vi "test-new-clock-3.vi"() -> ()   [LabVIEW 2019]
uses:
  <vilib>/Rock Robotics/WPI/ThirdParty/JAS_Junk/TrajLib/Trajectory_Library.lvlib
  <vilib>/Utility/RT CPU Load.ctl
panel:
  out "Overflow count":i32
  out "Loop5":i32
  out "Err Sum6":i32
  out "Clock6":dbl
  out "Err Sum5":i32
  out "Clock5":dbl
  out "RoboRIO CPU loads":T1[](array[typedef]) {"ISR (%)" format="%#.2f"; "Idle (%)" format="%#.2f"; "Background (%)" format="%#.2f"; "Normal (%)" format="%#.2f"; "Above Normal (%)" format="%#.2f"; "High (%)" format="%#.2g"; "Timed Structures (%)" format="%#.2g"; "Time Critical (%)" format="%#.2g"; "Total (%)" format="%#.2g"}
  out "Diff":dbl
  out "Err Sum4":i32
  out "Clock4":dbl
  out "Err Sum3":i32
  out "Clock3":dbl
  out "Err Sum2":i32
  out "Clock2":dbl
  out "Clock1":dbl
  out "Err Sum1":i32
  out "OS Clock":dbl format="%35.6f"
  out "Error Count":i32
  out "Loop Count":i32
  out "FPGA Clock":dbl format="%35.6f"
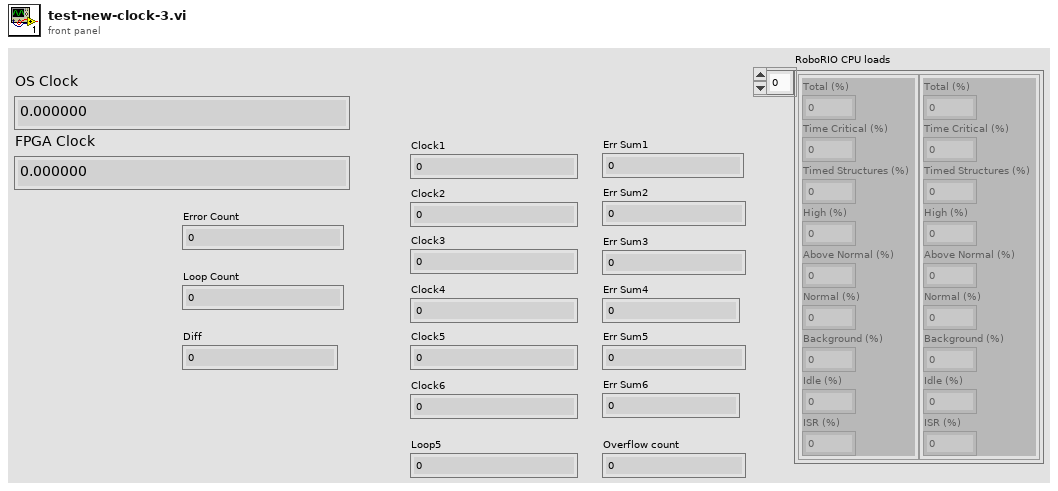
[diagram p1: front panel]
types:
  T1 = typedef "NI_Real-Time Target Support.lvlib/RT CPU Load.ctl" = cluster{"Total (%)":dbl, "Time Critical (%)":dbl, "Timed Structures (%)":dbl, "High (%)":dbl, "Above Normal (%)":dbl, "Normal (%)":dbl, "Background (%)":dbl, "Idle (%)":dbl, "ISR (%)":dbl}
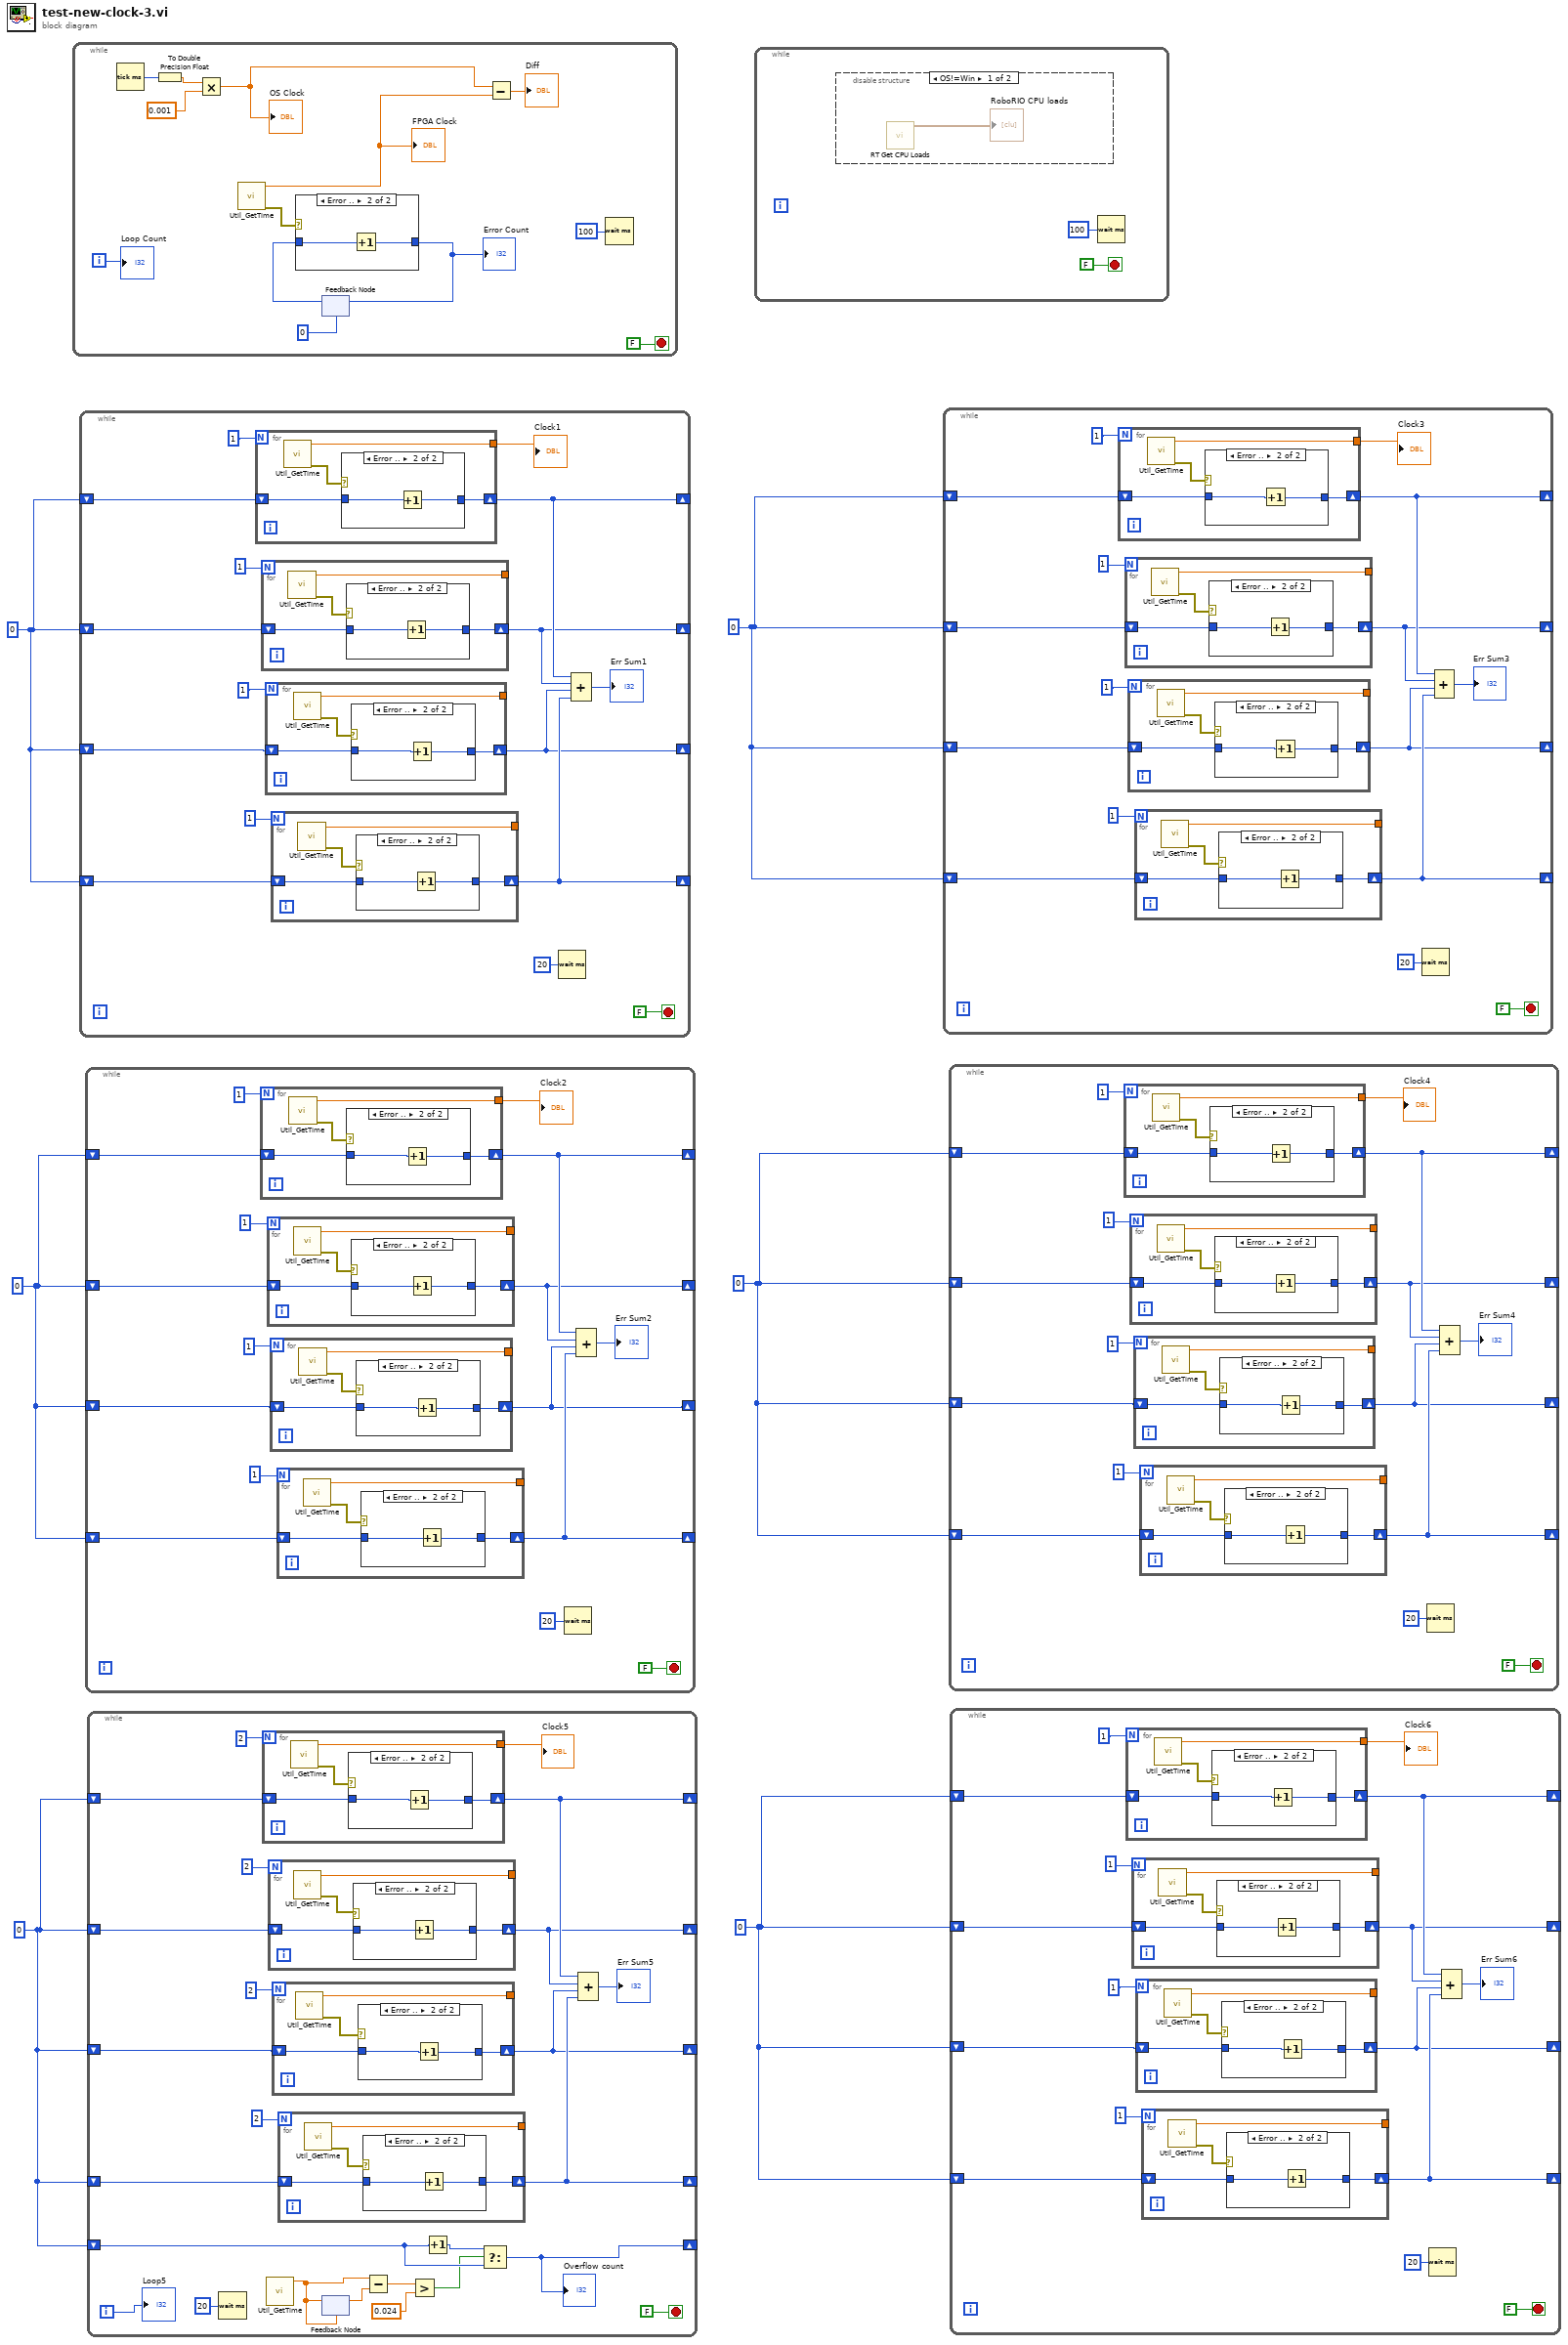
[diagram p0: block diagram]
diagram:
  w2 = 0
  w1 = 0
  w3 = 0
  w4 = 0
  w5 = 0
  w6 = 0
  n1 = while {
    i -> [w18]
    stop <- FALSE stop-if-true
    n2 = Tick Count (ms)() -> (millisecond timer value=w12:u32)
    n3 = To Double Precision Float(number=w12) -> (double precision float=w11:dbl)
    n4 = Multiply(x=w11, y=0.001) -> (x*y=w9:dbl)
    "OS Clock" <- w9
    n5 = call <vilib>:"Util_GetTime.vi"() -> ("error out"=w16:errorcluster, "FPGA_Time_Seconds"=w8:dbl)  [unwired: 10 in]
    "FPGA Clock" <- w8
    n6 = feedback #1(0) -> (w15:i32)
    n7 = case shown="Error .." w16 {
      tunnel: w15 -> [w20 w21]
      tunnel: [w20 w22] -> w14
      frame No Error {
      }
      frame Error {
        n8 = Increment(x=w21) -> (x+1=w22:i32)
      }
    }
    "Error Count" <- w14
    n9 = feedback-in #1(w14) -> ()
    n10 = Subtract(x=w9, y=w8) -> (x-y=→"Diff":dbl)
    n11 = Wait (ms)(milliseconds to wait=u32 100) -> ()  [unwired: 1 out]
    "Loop Count" <- w18
  }
  n12 = while {
    shift-right: [w27] -> _
    shift-left: w6 -> [w34]
    shift-right: [w28] -> _
    shift-left: w6 -> [w33]
    shift-right: [w25] -> _
    shift-left: w6 -> [w30]
    shift-right: [w26] -> _
    shift-left: w6 -> [w29]
    stop <- FALSE stop-if-true
    n13 = for {
      N: 1 -> [_]
      shift-right: [w61] -> w28
      shift-left: w33 -> [w62]
      tunnel: [w60] -> w23
      n14 = call <vilib>:"Util_GetTime.vi"() -> ("error out"=w63:errorcluster, "FPGA_Time_Seconds"=w60:dbl)  [unwired: 10 in]
      n15 = case shown="Error .." w63 {
        tunnel: [w64 w66] -> w61
        tunnel: w62 -> [w64 w65]
        frame No Error {
        }
        frame Error {
          n16 = Increment(x=w65) -> (x+1=w66:i32)
        }
      }
    }
    "Clock1" <- w23
    n17 = for {
      N: 1 -> [_]
      shift-right: [w54] -> w27
      shift-left: w34 -> [w55]
      tunnel: [w53] -> _
      n18 = call <vilib>:"Util_GetTime.vi"() -> ("error out"=w56:errorcluster, "FPGA_Time_Seconds"=w53:dbl)  [unwired: 10 in]
      n19 = case shown="Error .." w56 {
        tunnel: [w57 w59] -> w54
        tunnel: w55 -> [w57 w58]
        frame No Error {
        }
        frame Error {
          n20 = Increment(x=w58) -> (x+1=w59:i32)
        }
      }
    }
    n21 = for {
      N: 1 -> [_]
      shift-right: [w47] -> w25
      shift-left: w30 -> [w48]
      tunnel: [w46] -> _
      n22 = call <vilib>:"Util_GetTime.vi"() -> ("error out"=w49:errorcluster, "FPGA_Time_Seconds"=w46:dbl)  [unwired: 10 in]
      n23 = case shown="Error .." w49 {
        tunnel: [w50 w52] -> w47
        tunnel: w48 -> [w50 w51]
        frame No Error {
        }
        frame Error {
          n24 = Increment(x=w51) -> (x+1=w52:i32)
        }
      }
    }
    n25 = for {
      N: 1 -> [_]
      shift-right: [w40] -> w26
      shift-left: w29 -> [w41]
      tunnel: [w39] -> _
      n26 = call <vilib>:"Util_GetTime.vi"() -> ("error out"=w42:errorcluster, "FPGA_Time_Seconds"=w39:dbl)  [unwired: 10 in]
      n27 = case shown="Error .." w42 {
        tunnel: [w43 w45] -> w40
        tunnel: w41 -> [w43 w44]
        frame No Error {
        }
        frame Error {
          n28 = Increment(x=w44) -> (x+1=w45:i32)
        }
      }
    }
    n29 = Wait (ms)(milliseconds to wait=u32 20) -> ()  [unwired: 1 out]
    n30 = Compound Arithmetic op=ADD(w28, w27, w25, w26) -> (→"Err Sum1":i32)
  }
  n31 = while {
    shift-right: [w71] -> _
    shift-left: w5 -> [w78]
    shift-right: [w72] -> _
    shift-left: w5 -> [w77]
    shift-right: [w69] -> _
    shift-left: w5 -> [w74]
    shift-right: [w70] -> _
    shift-left: w5 -> [w73]
    stop <- FALSE stop-if-true
    n32 = for {
      N: 1 -> [_]
      shift-right: [w105] -> w72
      shift-left: w77 -> [w106]
      tunnel: [w104] -> w67
      n33 = call <vilib>:"Util_GetTime.vi"() -> ("error out"=w107:errorcluster, "FPGA_Time_Seconds"=w104:dbl)  [unwired: 10 in]
      n34 = case shown="Error .." w107 {
        tunnel: [w108 w110] -> w105
        tunnel: w106 -> [w108 w109]
        frame No Error {
        }
        frame Error {
          n35 = Increment(x=w109) -> (x+1=w110:i32)
        }
      }
    }
    "Clock2" <- w67
    n36 = for {
      N: 1 -> [_]
      shift-right: [w98] -> w71
      shift-left: w78 -> [w99]
      tunnel: [w97] -> _
      n37 = call <vilib>:"Util_GetTime.vi"() -> ("error out"=w100:errorcluster, "FPGA_Time_Seconds"=w97:dbl)  [unwired: 10 in]
      n38 = case shown="Error .." w100 {
        tunnel: [w101 w103] -> w98
        tunnel: w99 -> [w101 w102]
        frame No Error {
        }
        frame Error {
          n39 = Increment(x=w102) -> (x+1=w103:i32)
        }
      }
    }
    n40 = for {
      N: 1 -> [_]
      shift-right: [w91] -> w69
      shift-left: w74 -> [w92]
      tunnel: [w90] -> _
      n41 = call <vilib>:"Util_GetTime.vi"() -> ("error out"=w93:errorcluster, "FPGA_Time_Seconds"=w90:dbl)  [unwired: 10 in]
      n42 = case shown="Error .." w93 {
        tunnel: [w94 w96] -> w91
        tunnel: w92 -> [w94 w95]
        frame No Error {
        }
        frame Error {
          n43 = Increment(x=w95) -> (x+1=w96:i32)
        }
      }
    }
    n44 = for {
      N: 1 -> [_]
      shift-right: [w84] -> w70
      shift-left: w73 -> [w85]
      tunnel: [w83] -> _
      n45 = call <vilib>:"Util_GetTime.vi"() -> ("error out"=w86:errorcluster, "FPGA_Time_Seconds"=w83:dbl)  [unwired: 10 in]
      n46 = case shown="Error .." w86 {
        tunnel: [w87 w89] -> w84
        tunnel: w85 -> [w87 w88]
        frame No Error {
        }
        frame Error {
          n47 = Increment(x=w88) -> (x+1=w89:i32)
        }
      }
    }
    n48 = Wait (ms)(milliseconds to wait=u32 20) -> ()  [unwired: 1 out]
    n49 = Compound Arithmetic op=ADD(w72, w71, w69, w70) -> (→"Err Sum2":i32)
  }
  n50 = while {
    shift-right: [w124] -> _
    shift-left: w1 -> [w131]
    shift-right: [w125] -> _
    shift-left: w1 -> [w130]
    shift-right: [w122] -> _
    shift-left: w1 -> [w127]
    shift-right: [w123] -> _
    shift-left: w1 -> [w126]
    shift-right: [w112] -> _
    shift-left: w1 -> [w114]
    i -> [w119]
    stop <- FALSE stop-if-true
    n51 = Wait (ms)(milliseconds to wait=u32 20) -> ()  [unwired: 1 out]
    n52 = for {
      N: 2 -> [_]
      shift-right: [w158] -> w125
      shift-left: w130 -> [w159]
      tunnel: [w157] -> w120
      n53 = call <vilib>:"Util_GetTime.vi"() -> ("error out"=w160:errorcluster, "FPGA_Time_Seconds"=w157:dbl)  [unwired: 10 in]
      n54 = case shown="Error .." w160 {
        tunnel: [w161 w163] -> w158
        tunnel: w159 -> [w161 w162]
        frame No Error {
        }
        frame Error {
          n55 = Increment(x=w162) -> (x+1=w163:i32)
        }
      }
    }
    "Clock5" <- w120
    n56 = call <vilib>:"Util_GetTime.vi"() -> ("FPGA_Time_Seconds"=w117:dbl)  [unwired: 10 in, 1 out]
    n57 = for {
      N: 2 -> [_]
      shift-right: [w152] -> w124
      shift-left: w131 -> [w153]
      tunnel: [w151] -> _
      n58 = call <vilib>:"Util_GetTime.vi"() -> ("error out"=w150:errorcluster, "FPGA_Time_Seconds"=w151:dbl)  [unwired: 10 in]
      n59 = case shown="Error .." w150 {
        tunnel: [w154 w156] -> w152
        tunnel: w153 -> [w154 w155]
        frame No Error {
        }
        frame Error {
          n60 = Increment(x=w155) -> (x+1=w156:i32)
        }
      }
    }
    n61 = for {
      N: 2 -> [_]
      shift-right: [w145] -> w122
      shift-left: w127 -> [w146]
      tunnel: [w144] -> _
      n62 = call <vilib>:"Util_GetTime.vi"() -> ("error out"=w143:errorcluster, "FPGA_Time_Seconds"=w144:dbl)  [unwired: 10 in]
      n63 = case shown="Error .." w143 {
        tunnel: [w147 w149] -> w145
        tunnel: w146 -> [w147 w148]
        frame No Error {
        }
        frame Error {
          n64 = Increment(x=w148) -> (x+1=w149:i32)
        }
      }
    }
    n65 = for {
      N: 2 -> [_]
      shift-right: [w138] -> w123
      shift-left: w126 -> [w139]
      tunnel: [w137] -> _
      n66 = call <vilib>:"Util_GetTime.vi"() -> ("error out"=w136:errorcluster, "FPGA_Time_Seconds"=w137:dbl)  [unwired: 10 in]
      n67 = case shown="Error .." w136 {
        tunnel: [w140 w142] -> w138
        tunnel: w139 -> [w140 w141]
        frame No Error {
        }
        frame Error {
          n68 = Increment(x=w141) -> (x+1=w142:i32)
        }
      }
    }
    n69 = feedback-in #2(w117) -> ()
    n70 = feedback #2(w117) -> (w118:dbl)
    n71 = Subtract(x=w117, y=w118) -> (x-y=w116:dbl)
    n72 = Greater?(x=w116, y=0.024) -> (0:w111:bool)
    n73 = Increment(x=w114) -> (x+1=w113:i32)
    n74 = Select(t=w113, s=w111, f=w114) -> (s? t:f=w112:i32)
    "Overflow count" <- w112
    n75 = Compound Arithmetic op=ADD(w125, w124, w122, w123) -> (→"Err Sum5":i32)
    "Loop5" <- w119
  }
  n76 = while {
    stop <- FALSE stop-if-true
    n77 = disable-structure shown="OS!=Win" {
      frame condition #0 {
        n78 = call <vilib>:"RT Get CPU Loads.vi"() -> ("CPU loads"=→"RoboRIO CPU loads":T1[])  [unwired: 10 in, 1 out]
      }
      frame condition #1 (active) {
      }
    }
    n79 = Wait (ms)(milliseconds to wait=u32 100) -> ()  [unwired: 1 out]
  }
  n80 = while {
    shift-right: [w171] -> _
    shift-left: w4 -> [w178]
    shift-right: [w172] -> _
    shift-left: w4 -> [w177]
    shift-right: [w169] -> _
    shift-left: w4 -> [w174]
    shift-right: [w170] -> _
    shift-left: w4 -> [w173]
    stop <- FALSE stop-if-true
    n81 = for {
      N: 1 -> [_]
      shift-right: [w205] -> w172
      shift-left: w177 -> [w206]
      tunnel: [w204] -> w167
      n82 = call <vilib>:"Util_GetTime.vi"() -> ("error out"=w207:errorcluster, "FPGA_Time_Seconds"=w204:dbl)  [unwired: 10 in]
      n83 = case shown="Error .." w207 {
        tunnel: [w208 w210] -> w205
        tunnel: w206 -> [w208 w209]
        frame No Error {
        }
        frame Error {
          n84 = Increment(x=w209) -> (x+1=w210:i32)
        }
      }
    }
    "Clock3" <- w167
    n85 = for {
      N: 1 -> [_]
      shift-right: [w198] -> w171
      shift-left: w178 -> [w199]
      tunnel: [w197] -> _
      n86 = call <vilib>:"Util_GetTime.vi"() -> ("error out"=w200:errorcluster, "FPGA_Time_Seconds"=w197:dbl)  [unwired: 10 in]
      n87 = case shown="Error .." w200 {
        tunnel: [w201 w203] -> w198
        tunnel: w199 -> [w201 w202]
        frame No Error {
        }
        frame Error {
          n88 = Increment(x=w202) -> (x+1=w203:i32)
        }
      }
    }
    n89 = for {
      N: 1 -> [_]
      shift-right: [w191] -> w169
      shift-left: w174 -> [w192]
      tunnel: [w190] -> _
      n90 = call <vilib>:"Util_GetTime.vi"() -> ("error out"=w193:errorcluster, "FPGA_Time_Seconds"=w190:dbl)  [unwired: 10 in]
      n91 = case shown="Error .." w193 {
        tunnel: [w194 w196] -> w191
        tunnel: w192 -> [w194 w195]
        frame No Error {
        }
        frame Error {
          n92 = Increment(x=w195) -> (x+1=w196:i32)
        }
      }
    }
    n93 = for {
      N: 1 -> [_]
      shift-right: [w184] -> w170
      shift-left: w173 -> [w185]
      tunnel: [w183] -> _
      n94 = call <vilib>:"Util_GetTime.vi"() -> ("error out"=w186:errorcluster, "FPGA_Time_Seconds"=w183:dbl)  [unwired: 10 in]
      n95 = case shown="Error .." w186 {
        tunnel: [w187 w189] -> w184
        tunnel: w185 -> [w187 w188]
        frame No Error {
        }
        frame Error {
          n96 = Increment(x=w188) -> (x+1=w189:i32)
        }
      }
    }
    n97 = Wait (ms)(milliseconds to wait=u32 20) -> ()  [unwired: 1 out]
    n98 = Compound Arithmetic op=ADD(w172, w171, w169, w170) -> (→"Err Sum3":i32)
  }
  n99 = while {
    shift-right: [w215] -> _
    shift-left: w3 -> [w222]
    shift-right: [w216] -> _
    shift-left: w3 -> [w221]
    shift-right: [w213] -> _
    shift-left: w3 -> [w218]
    shift-right: [w214] -> _
    shift-left: w3 -> [w217]
    stop <- FALSE stop-if-true
    n100 = for {
      N: 1 -> [_]
      shift-right: [w249] -> w216
      shift-left: w221 -> [w250]
      tunnel: [w248] -> w211
      n101 = call <vilib>:"Util_GetTime.vi"() -> ("error out"=w251:errorcluster, "FPGA_Time_Seconds"=w248:dbl)  [unwired: 10 in]
      n102 = case shown="Error .." w251 {
        tunnel: [w252 w254] -> w249
        tunnel: w250 -> [w252 w253]
        frame No Error {
        }
        frame Error {
          n103 = Increment(x=w253) -> (x+1=w254:i32)
        }
      }
    }
    "Clock4" <- w211
    n104 = for {
      N: 1 -> [_]
      shift-right: [w242] -> w215
      shift-left: w222 -> [w243]
      tunnel: [w241] -> _
      n105 = call <vilib>:"Util_GetTime.vi"() -> ("error out"=w244:errorcluster, "FPGA_Time_Seconds"=w241:dbl)  [unwired: 10 in]
      n106 = case shown="Error .." w244 {
        tunnel: [w245 w247] -> w242
        tunnel: w243 -> [w245 w246]
        frame No Error {
        }
        frame Error {
          n107 = Increment(x=w246) -> (x+1=w247:i32)
        }
      }
    }
    n108 = for {
      N: 1 -> [_]
      shift-right: [w235] -> w213
      shift-left: w218 -> [w236]
      tunnel: [w234] -> _
      n109 = call <vilib>:"Util_GetTime.vi"() -> ("error out"=w237:errorcluster, "FPGA_Time_Seconds"=w234:dbl)  [unwired: 10 in]
      n110 = case shown="Error .." w237 {
        tunnel: [w238 w240] -> w235
        tunnel: w236 -> [w238 w239]
        frame No Error {
        }
        frame Error {
          n111 = Increment(x=w239) -> (x+1=w240:i32)
        }
      }
    }
    n112 = for {
      N: 1 -> [_]
      shift-right: [w228] -> w214
      shift-left: w217 -> [w229]
      tunnel: [w227] -> _
      n113 = call <vilib>:"Util_GetTime.vi"() -> ("error out"=w230:errorcluster, "FPGA_Time_Seconds"=w227:dbl)  [unwired: 10 in]
      n114 = case shown="Error .." w230 {
        tunnel: [w231 w233] -> w228
        tunnel: w229 -> [w231 w232]
        frame No Error {
        }
        frame Error {
          n115 = Increment(x=w232) -> (x+1=w233:i32)
        }
      }
    }
    n116 = Wait (ms)(milliseconds to wait=u32 20) -> ()  [unwired: 1 out]
    n117 = Compound Arithmetic op=ADD(w216, w215, w213, w214) -> (→"Err Sum4":i32)
  }
  n118 = while {
    shift-right: [w259] -> _
    shift-left: w2 -> [w266]
    shift-right: [w260] -> _
    shift-left: w2 -> [w265]
    shift-right: [w257] -> _
    shift-left: w2 -> [w262]
    shift-right: [w258] -> _
    shift-left: w2 -> [w261]
    stop <- FALSE stop-if-true
    n119 = for {
      N: 1 -> [_]
      shift-right: [w293] -> w260
      shift-left: w265 -> [w294]
      tunnel: [w292] -> w255
      n120 = call <vilib>:"Util_GetTime.vi"() -> ("error out"=w295:errorcluster, "FPGA_Time_Seconds"=w292:dbl)  [unwired: 10 in]
      n121 = case shown="Error .." w295 {
        tunnel: [w296 w298] -> w293
        tunnel: w294 -> [w296 w297]
        frame No Error {
        }
        frame Error {
          n122 = Increment(x=w297) -> (x+1=w298:i32)
        }
      }
    }
    "Clock6" <- w255
    n123 = for {
      N: 1 -> [_]
      shift-right: [w286] -> w259
      shift-left: w266 -> [w287]
      tunnel: [w285] -> _
      n124 = call <vilib>:"Util_GetTime.vi"() -> ("error out"=w288:errorcluster, "FPGA_Time_Seconds"=w285:dbl)  [unwired: 10 in]
      n125 = case shown="Error .." w288 {
        tunnel: [w289 w291] -> w286
        tunnel: w287 -> [w289 w290]
        frame No Error {
        }
        frame Error {
          n126 = Increment(x=w290) -> (x+1=w291:i32)
        }
      }
    }
    n127 = for {
      N: 1 -> [_]
      shift-right: [w279] -> w257
      shift-left: w262 -> [w280]
      tunnel: [w278] -> _
      n128 = call <vilib>:"Util_GetTime.vi"() -> ("error out"=w281:errorcluster, "FPGA_Time_Seconds"=w278:dbl)  [unwired: 10 in]
      n129 = case shown="Error .." w281 {
        tunnel: [w282 w284] -> w279
        tunnel: w280 -> [w282 w283]
        frame No Error {
        }
        frame Error {
          n130 = Increment(x=w283) -> (x+1=w284:i32)
        }
      }
    }
    n131 = for {
      N: 1 -> [_]
      shift-right: [w272] -> w258
      shift-left: w261 -> [w273]
      tunnel: [w271] -> _
      n132 = call <vilib>:"Util_GetTime.vi"() -> ("error out"=w274:errorcluster, "FPGA_Time_Seconds"=w271:dbl)  [unwired: 10 in]
      n133 = case shown="Error .." w274 {
        tunnel: [w275 w277] -> w272
        tunnel: w273 -> [w275 w276]
        frame No Error {
        }
        frame Error {
          n134 = Increment(x=w276) -> (x+1=w277:i32)
        }
      }
    }
    n135 = Wait (ms)(milliseconds to wait=u32 20) -> ()  [unwired: 1 out]
    n136 = Compound Arithmetic op=ADD(w260, w259, w257, w258) -> (→"Err Sum6":i32)
  }
